vi "Do.vi"(8 "error in (no error)":errorcluster, 10 "Actor in":refnum<class "Actor.lvclass">, 11 "Write game board Msg":refnum<class "Write game board Msg.lvclass">) -> (0 "error out":errorcluster, 2 "Actor out":refnum<class "Actor.lvclass">)   [LabVIEW 2014, in "GoBang.lvlib" / "Write game board Msg.lvclass"]
doc: "This VI delivers the message to the actor by calling the appropriate method(s) on the actor."
uses:
  Write game board Msg.lvclass
  Client/CS++GoBangClient.lvclass
  CSPP_Core/Actors/CS++PVMonitor Messages/CS++PVUpdate Msg/CS++PVUpdate Msg.lvclass
  CSPP_Core/Classes/CS++ProcessVariables/ProcessVariable/PV.lvclass
  <vilib>/ActorFramework/Actor/Actor.lvclass
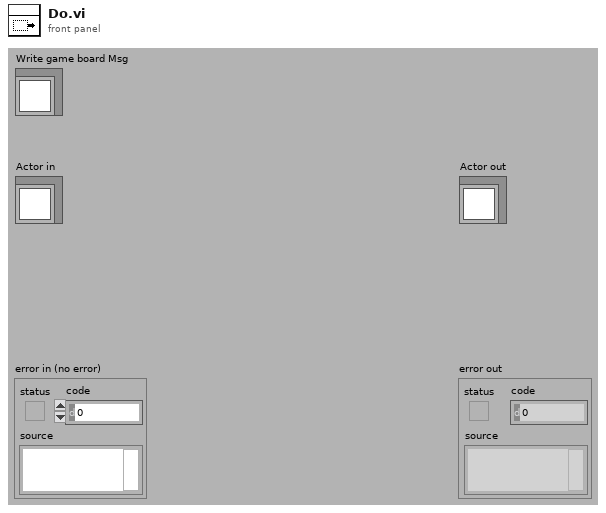
[diagram p1: front panel]
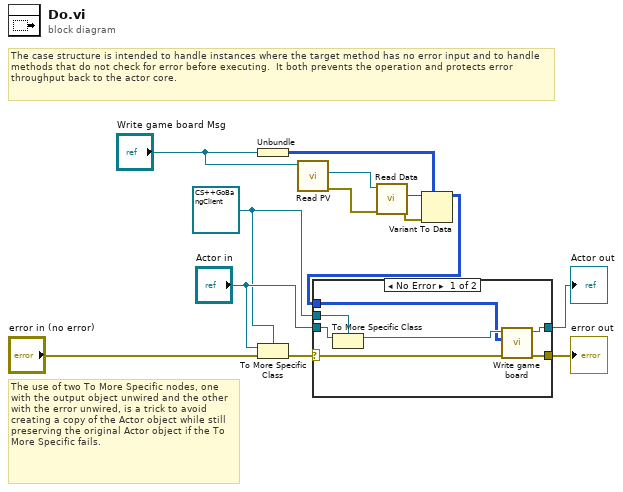
[diagram p0: block diagram]
diagram:
  w8 = refnum<class "CS++GoBangClient.lvclass"> refnum ("Actor in")
  # "The use of two To More Specific nodes, one with the output object unwired and the other with the error unwired, is a trick to avoid creating a copy of the Actor object while still preserving the original Actor object if the To More Specific fails."
  # "The case structure is intended to handle instances where the target method has no error input and to handle methods that do not check for error before executing.  It both prevents the operation and protects error throughput back to the actor core."
  n1 = Unbundle("Write game board Msg") -> (w3:u8[][])
  n2 = To More Specific Class(target class=w8, reference="Actor in", error in="error in (no error)") -> (error out=w12:errorcluster)  [unwired: 1 out]
  n3 = call "Read PV.vi"("CS++PVUpdate Msg in"="Write game board Msg") -> ("error out"=w4:errorcluster, "PV"=w5:refnum<class "PV.lvclass">)  [unwired: 8 in, 1 out]
  n4 = call "Read Data.vi"("error in (no error)"=w4, "PV in"=w5) -> ("error out"=w6:errorcluster, "Data"=w7:variant)  [unwired: 7 in, 1 out]
  n5 = Variant To Data(error in=w6, type=w3, Variant=w7) -> (data=w1:u8[][])  [unwired: 1 out]
  n6 = case shown="No Error" w12 {
    selector: w12 -> [w18 w22]
    tunnel: [w20 w22] -> w11
    tunnel: [w19 w21] -> w10
    tunnel: "Actor in" -> [w17 w21]
    tunnel: w8 -> [w16 _]
    tunnel: w1 -> [w14 _]
    frame No Error {
      n7 = To More Specific Class(target class=w16, reference=w17) -> (specific class reference=w15:refnum<class "CS++GoBangClient.lvclass">)  [unwired: 1 in, 1 out]
      n8 = call-dynamic "Write game board.vi"("error in (no error)"=w18, "GameBoard"=w14, "CS++GoBangClient in"=w15) -> ("error out"=w20:errorcluster, "CS++GoBangClient out"=w19:refnum<class "CS++GoBangClient.lvclass">)  [unwired: 7 in]
    }
    frame Error {
      # "If type check fails, pass the original object out again."
    }
  }
  "error out" <- w11
  "Actor out" <- w10
